vi "Fetch Multi Eval Meas ES Flatness Subcarrier Index Results.vi"(8 "error in (no error)":errorcluster, 10 "Instance (1)":T2=1, 11 "VISA resource name":refnum<visa-resource-name>) -> (0 "error out":errorcluster, 1 "Subcarrier Index Results":T1, 2 "Reliability":i32, 3 "VISA resource name out":refnum<visa-resource-name>, 5 "Out Of Tolerance":i32)   [LabVIEW 2020, in "Rohde&Schwarz CMWXP NR FR1 Measurement.lvlib"]
doc: "Returns subcarrier indices of the equalizer spectrum flatness measurement. At these SC indices, the current minimum and maximum power of the equalizer coefficients have been detected within range 1 and range 2.\n\nAttribute:\nRSCMWXPNRFR1M_ATTR_FETCH_MULTI_EVAL_MEAS_ES_FLATNESS_SUBCARRIER_INDEX_RESULTS\n\nRemote-control command:\nFETCh:NRSub:MEAS<i>:MEValuation:ESFLatness:CURRent:SCINdex?"
uses:
  <instrlib>/Rohde&Schwarz CMWXP NR FR1 Measurement/Rohde&Schwarz CMWXP NR FR1 Measurement.lvlib
  <instrlib>/Rohde&Schwarz CMWXP NR FR1 Measurement/Private/_Instance.ctl
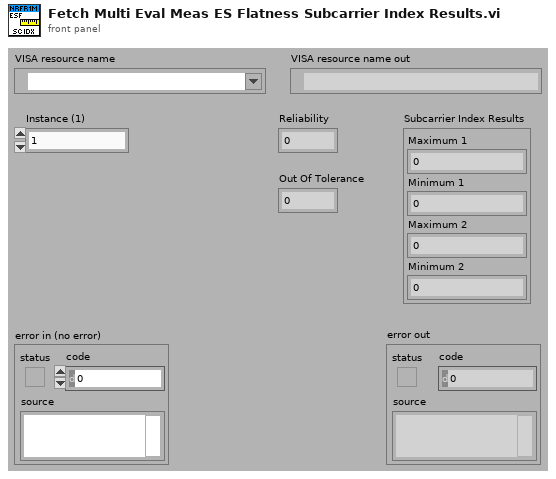
[diagram p1: front panel]
types:
  T1 = cluster{"Maximum 1":i32, "Minimum 1":i32, "Maximum 2":i32, "Minimum 2":i32}
  T2 = typedef "Rohde&Schwarz CMWXP NR FR1 Measurement.lvlib/_Instance.ctl" = i32
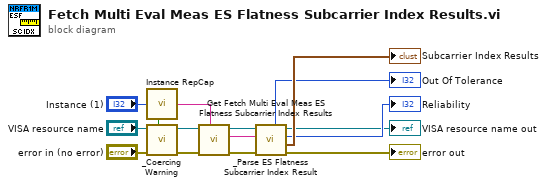
[diagram p0: block diagram]
diagram:
  n1 = call <instrlib>:"Instance RepCap.vi"("Instance In"="Instance (1)") -> ("In Range?"=w12:bool, "RepCap Identifier Out"=w11:string)  [unwired: 1 in]
  n2 = call <instrlib>:"_Coercing Warning.vi"("In Range?"=w12, "error in (no error)"="error in (no error)", "VISA resource name"="VISA resource name") -> ("error out"=w9:errorcluster, "VISA resource name out"=w10:refnum<visa-resource-name>)  [unwired: 7 in]
  n3 = call "Get Fetch Multi Eval Meas ES Flatness Subcarrier Index Results"("Repeated Capabilities"=w11, "error in (no error)"=w9, "instrument handle"=w10) -> ("error out"=w8:errorcluster, "Fetch Multi Eval Meas ES Flatness Subcarrier Index Results"=w7:string, "instrument handle out"=w6:refnum<visa-resource-name>)  [unwired: 6 in]
  n4 = call <instrlib>:"_Parse ES Flatness Subcarrier Index Result.vi"("error in (no error)"=w8, "Input String"=w7, "VISA resource name"=w6) -> ("error out"=→"error out":errorcluster, "Subcarrier Index Results"=→"Subcarrier Index Results":T1, "Reliability"=→"Reliability":i32, "VISA resource name out"=→"VISA resource name out":refnum<visa-resource-name>, "Out Of Tolerance"=→"Out Of Tolerance":i32)  [unwired: 4 in]
